vi "Auton File Control.vi"() -> ()   [LabVIEW 2017]
uses:
  Common Code/Utilities/Change Detect Boolean.vi
  Robot Global Data.vi
  Common Code/Utilities/Change Detect Int.vi
  Common Code/Gamepads/Button Cluster.ctl
  Common Code/Gamepads/D-Pad.ctl
panel:
  in  "D-Pad":T1
  in  "Button Cluster":T2
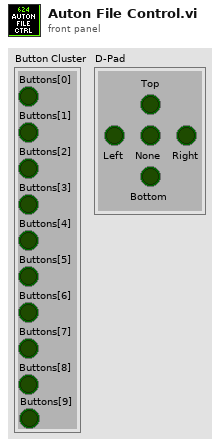
[diagram p1: front panel]
types:
  T1 = typedef "D-Pad.ctl" = cluster{"Top":bool, "Bottom":bool, "None":bool, "Right":bool, "Left":bool}
  T2 = typedef "Button Cluster.ctl" = cluster{"Buttons[0]":bool, "Buttons[1]":bool, "Buttons[2]":bool, "Buttons[3]":bool, "Buttons[4]":bool, "Buttons[5]":bool, "Buttons[6]":bool, "Buttons[7]":bool, "Buttons[8]":bool, "Buttons[9]":bool}
  T3 = typedef "Dashboard Control Data.ctl" = cluster{"Drivetrain Settings Cluster":T4, "Intake Presets":T6, "Elevator Settings Cluster":T7, "Drivetrain Encoder Values":T9, "Auton Chooser":T10}
  T4 = typedef "Drivetrain Settings Cluster.ctl" = cluster{"Gyro Steer PID Gains":T5, "Distance Drive PID Gains":T5, "Drive Tolerance":dbl, "Gyro Tolerance":dbl, "Gyro Output":dbl, "Distance Output":dbl, "Y Power Multiplier":dbl, "Turn Power Multiplier":dbl, "Creep Rate":dbl, "Constant Power":bool, "DT Mode Modifier":enum16{"None, Default", "Cube", "Square"}, "Left Encoder Tick Constant":dbl, "Right Encoder Tick Constant":dbl, "Shift Speed":dbl}
  T5 = typedef "PID Gains Cluster.ctl" = cluster{"Integral Time":dbl, "Proportional Gain":dbl, "Derivative Time":dbl}
  T6 = typedef "Intake Presets.ctl" = cluster{"Idle Angle":dbl, "Mid Angle":dbl, "Low Angle":dbl, "Outtake Power":dbl, "Intake Power":dbl, "Unstuck":dbl, "Angle Tolerance":dbl, "Max Angle":dbl, "Max Current":dbl, "Current Trip Time":dbl, "Reset Encoder?":bool, "Encoder Scale":dbl, "PID gains":cluster{"proportional gain (Kc)":dbl, "integral time (Ti, min)":dbl, "derivative time (Td, min)":dbl}, "output range":cluster{"output high":dbl, "output low":dbl}}
  T7 = typedef "Elevator Settings Cluster.ctl" = cluster{"Ground Height":dbl, "Switch Height":dbl, "Scale High Height ":dbl, "Scale Low Height":dbl, "Elevator PID Gains":T8, "Elevator Tolerance":dbl, "Reset Encoders":bool, "Encoder Scale":dbl, "Max Height":dbl, "Mid Height":dbl, "output range":cluster{"output high":dbl, "output low":dbl}, "Slow Down Tolerance":dbl}
  T8 = typedef "PID Gains.ctl" = cluster{"proportional gain (Kc)":dbl, "integral time (Ti, min)":dbl, "derivative time (Td, min)":dbl}
  T9 = typedef "DT Encoder Values.ctl" = cluster{"Left Encoder":cluster{"Distance":dbl, "Speed":dbl, "Tick":dbl}, "Right Encoder":cluster{"Distance":dbl, "Speed":dbl, "Tick":dbl}}
  T10 = typedef "Auton Chooser.ctl" = cluster{"Left":bool, "Center":bool, "Right":bool, "Scale":bool, "Both":bool, "Switch":bool, "Near":bool, "Far":bool}
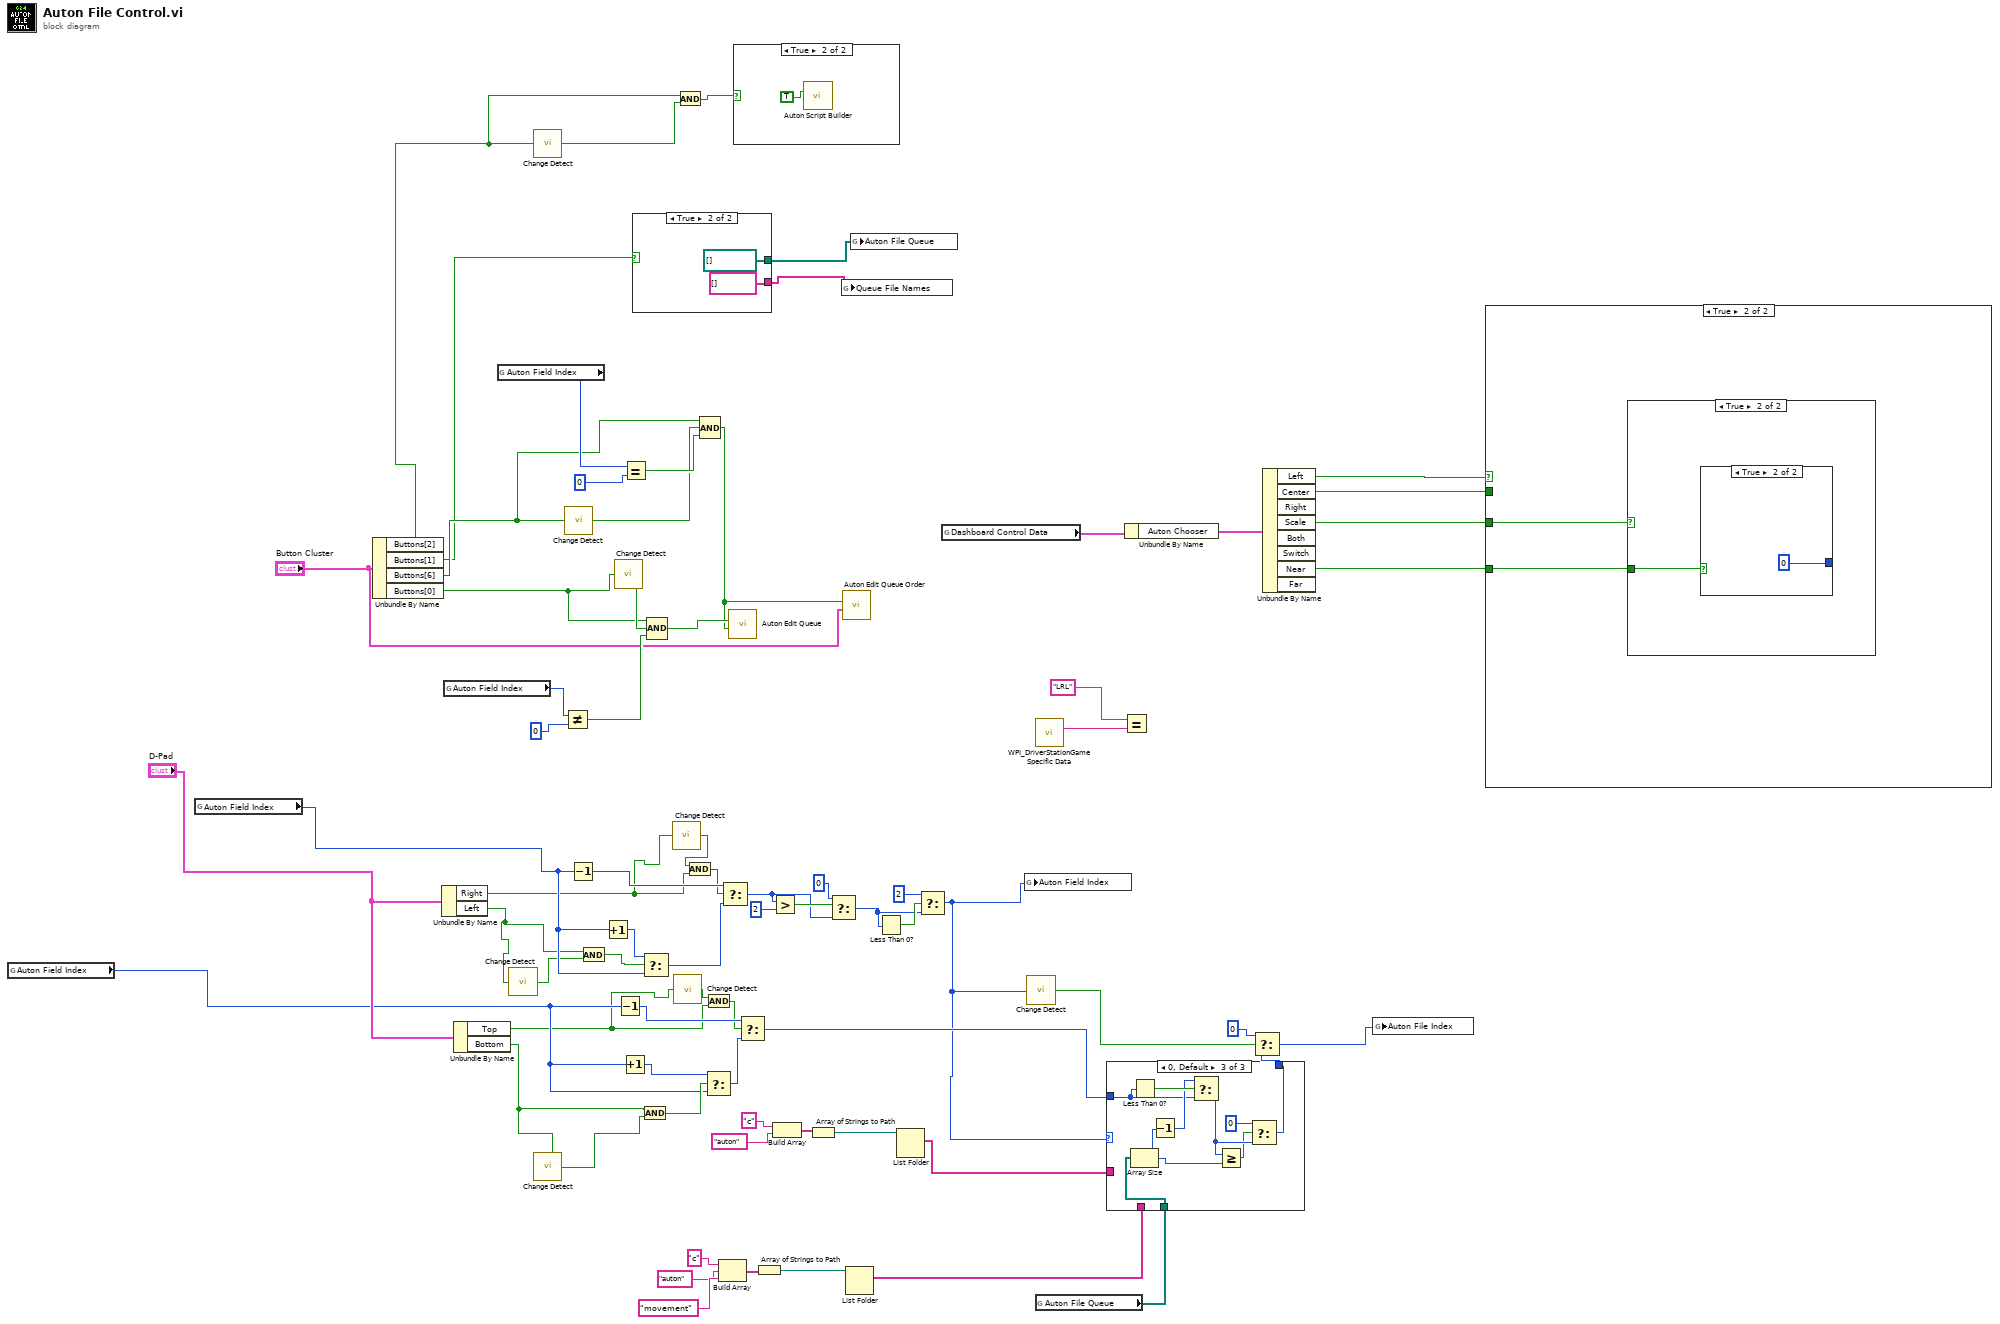
[diagram p0: block diagram]
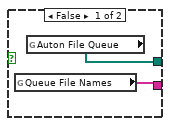
[diagram p6: hidden frame]
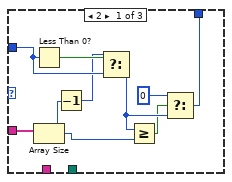
[diagram p8: hidden frame]
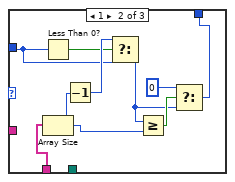
[diagram p9: hidden frame]
diagram:
  n1 = global read "Robot Global Data.vi" "Auton Field Index"() -> (w37:i32)
  n2 = global read "Robot Global Data.vi" "Auton Field Index"() -> (w38:i32)
  n3 = Unbundle By Name("Button Cluster") -> ("Buttons[2]"=w13:bool, "Buttons[1]"=w10:bool, "Buttons[6]"=w64:bool, "Buttons[0]"=w72:bool)
  n4 = Unbundle By Name("D-Pad") -> ("Right"=w29:bool, "Left"=w33:bool)
  n5 = global read "Robot Global Data.vi" "Auton Field Index"() -> (w71:i32)
  n6 = Unbundle By Name("D-Pad") -> ("Top"=w31:bool, "Bottom"=w36:bool)
  n7 = global read "Robot Global Data.vi" "Auton Field Index"() -> (w67:i32)
  n8 = call-poly "Change Detect.vi"("In"=w33) -> ("Changed?"=w34:bool)
  n9 = call-poly "Change Detect.vi"("In"=w13) -> ("Changed?"=w14:bool)
  n10 = call-poly "Change Detect.vi"("In"=w36) -> ("Changed?"=w35:bool)
  n11 = Not Equal?(x=w71, y=0) -> (x != y?=w69:bool)
  n12 = call-poly "Change Detect.vi"("In"=w64) -> ("Changed?"=w65:bool)
  n13 = Decrement(x=w38) -> (x-1=w60:i32)
  n14 = And(x=w33, y=w34) -> (x .and. y?=w42:bool)
  n15 = Increment(x=w38) -> (x+1=w59:i32)
  n16 = call-poly "Change Detect.vi"("In"=w72) -> ("Changed?"=w73:bool)
  n17 = Decrement(x=w37) -> (x-1=w48:i32)
  n18 = Increment(x=w37) -> (x+1=w49:i32)
  n19 = Equal?(x=w67, y=0) -> (x = y?=w66:bool)
  n20 = case shown="True" w10 {
    tunnel: [w75 path[] [] ("Auton File Queue")] -> w12
    tunnel: [w74 string[] [] ("Queue File Names")] -> w11
    frame False {
      n21 = global read "Robot Global Data.vi" "Queue File Names"() -> (w74:string[])
      n22 = global read "Robot Global Data.vi" "Auton File Queue"() -> (w75:path[])
    }
    frame True {
    }
  }
  n23 = And(x=w36, y=w35) -> (x .and. y?=w40:bool)
  n24 = Select(t=w59, s=w42, f=w38) -> (s? t:f=w58:i32)
  n25 = Compound Arithmetic op=AND(w72, w73, w69) -> (w63:bool)
  n26 = call-poly "Change Detect.vi"("In"=w29) -> ("Changed?"=w30:bool)
  n27 = call-poly "Change Detect.vi"("In"=w31) -> ("Changed?"=w32:bool)
  n28 = And(x=w13, y=w14) -> (x .and. y?=w15:bool)
  n29 = And(x=w30, y=w29) -> (x .and. y?=w43:bool)
  n30 = Compound Arithmetic op=AND(w64, w65, w66) -> (w62:bool)
  n31 = And(x=w32, y=w31) -> (x .and. y?=w41:bool)
  n32 = Select(t=w49, s=w40, f=w37) -> (s? t:f=w50:i32)
  n33 = Build Array("c", "auton", "movement" ("element")) -> (w26:string[])
  n34 = Select(t=w60, s=w43, f=w58) -> (s? t:f=w55:i32)
  n35 = call "Auton Edit Queue.vi"("Delete?"=w62, "Add?"=w63) -> ()  [unwired: 10 in]
  n36 = case shown="True" w15 {
    frame False {
    }
    frame True {
      n37 = call "Auton Script Builder.vi"("Export?"=TRUE) -> ()  [unwired: 10 in, 1 out]
    }
  }
  n38 = Select(t=w48, s=w41, f=w50) -> (s? t:f=w28:i32)
  n39 = Array of Strings to Path(0:w26) -> (2:w24:path)  [unwired: 1 in]
  n40 = Greater?(x=w55, y=2) -> (0:w56:bool)
  n41 = Build Array("c", "auton") -> (w46:string[])
  n42 = Array of Strings to Path(0:w46) -> (2:w44:path)  [unwired: 1 in]
  n43 = Select(t=0, s=w56, f=w55) -> (s? t:f=w52:i32)
  n44 = global write "Robot Global Data.vi" "Queue File Names"(w11) -> ()
  n45 = call "Auton Edit Queue Order.vi"("Button Cluster"="Button Cluster", "Boolean"=w62) -> ()  [unwired: 10 in]
  n46 = List Folder(path=w24) -> (filenames=w22:string[])  [unwired: 3 in, 3 out]
  n47 = global write "Robot Global Data.vi" "Auton File Queue"(w12) -> ()
  n48 = Less Than 0?(x=w52) -> (x < 0?=w53:bool)
  n49 = List Folder(path=w44) -> (filenames=w21:string[])  [unwired: 3 in, 3 out]
  n50 = Select(t=2, s=w53, f=w52) -> (s? t:f=w17:i32)
  n51 = global read "Robot Global Data.vi" "Dashboard Control Data"() -> (w8:T3)
  n52 = global write "Robot Global Data.vi" "Auton Field Index"(w17) -> ()
  n53 = call-poly "Change Detect.vi"("In"=w17) -> ("Changed?"=w18:bool)
  n54 = call <vilib>:"WPI_DriverStationGame Specific Data.vi"() -> ("Game Specific Data"=w2:string)  [unwired: 11 in]
  n55 = global read "Robot Global Data.vi" "Auton File Queue"() -> (w20:path[])
  n56 = case shown="0, Default" w17 {
    tunnel: w28 -> [w85 w89 w98]
    tunnel: w21 -> [w87 _ _]
    tunnel: w22 -> [_ w90 _]
    tunnel: w20 -> [_ _ w97]
    tunnel: [w79 w88 w99] -> w9
    frame 2 {
      n57 = Less Than 0?(x=w85) -> (x < 0?=w86:bool)
      n58 = Array Size(array=w87) -> (size(s)=w82:i32)
      n59 = Decrement(x=w82) -> (x-1=w84:i32)
      n60 = Select(t=w84, s=w86, f=w85) -> (s? t:f=w83:i32)
      n61 = Greater Or Equal?(x=w83, y=w82) -> (x >= y?=w81:bool)
      n62 = Select(t=0, s=w81, f=w83) -> (s? t:f=w79:i32)
    }
    frame 1 {
      n63 = Less Than 0?(x=w89) -> (x < 0?=w91:bool)
      n64 = Array Size(array=w90) -> (size(s)=w94:i32)
      n65 = Decrement(x=w94) -> (x-1=w92:i32)
      n66 = Select(t=w92, s=w91, f=w89) -> (s? t:f=w93:i32)
      n67 = Greater Or Equal?(x=w93, y=w94) -> (x >= y?=w95:bool)
      n68 = Select(t=0, s=w95, f=w93) -> (s? t:f=w88:i32)
    }
    frame 0, Default {
      n69 = Less Than 0?(x=w98) -> (x < 0?=w105:bool)
      n70 = Array Size(array=w97) -> (size(s)=w102:i32)
      n71 = Decrement(x=w102) -> (x-1=w104:i32)
      n72 = Select(t=w104, s=w105, f=w98) -> (s? t:f=w103:i32)
      n73 = Greater Or Equal?(x=w103, y=w102) -> (x >= y?=w101:bool)
      n74 = Select(t=0, s=w101, f=w103) -> (s? t:f=w99:i32)
    }
  }
  n75 = Equal?(x="LRL", y=w2) -> ()  [unwired: 1 out]
  n76 = Unbundle By Name(w8) -> ("Auton Chooser"=w7:T10)
  n77 = Select(t=0, s=w18, f=w9) -> (s? t:f=w16:i32)
  n78 = Unbundle By Name(w7) -> ("Left"=w6:bool, "Center"=w5:bool, "Scale"=w4:bool, "Near"=w3:bool)  [unwired: 4 out]
  n79 = global write "Robot Global Data.vi" "Auton File Index"(w16) -> ()
  n80 = case shown="True" w6 {
    tunnel: w5 -> [w106 _]
    tunnel: w4 -> [_ w108]
    tunnel: w3 -> [_ w107]
    frame False {
      n81 = case shown="True" w106 {
        frame False {
        }
        frame True {
        }
      }
    }
    frame True {
      n82 = case shown="True" w108 {
        tunnel: w107 -> [_ w109]
        frame False {
        }
        frame True {
          n83 = case shown="True" w109 {
            tunnel: [_ 0] -> _
            frame False {
            }
            frame True {
            }
          }
        }
      }
    }
  }
